vi "Tester.vi"() -> ()   [LabVIEW 2024]
uses:
  Shared Modules/CAN Commands Interpreter/CAN Frame Data.ctl
  Shared Modules/CAN Commands Interpreter/XNET Session Settings.ctl
  Type Definitions/Tester References.ctl
  Shared Modules/CAN Commands Interpreter/Command Values.ctl
  <vilib>/FPGAPlugInAG/PXI-7842R/niLvFpga_Open_PXI-7842R.vi
  <vilib>/rvi/interface/common/dynamic/niFpgaDynamicAddResources.vi
  <vilib>/FPGAPlugInAG/Dynamic/niLvFpga_Reset_Dynamic.vi
  Modules/Working Mode/Set Working Mode.vi
  Shared Modules/CAN Commands Interpreter/Target Sessions - Stop Session.vi
  Shared Modules/CAN Commands Interpreter/Target Sessions - Start Session.vi
  Shared Modules/CAN Commands Interpreter/Target Sessions - Clear Session.vi
  Shared Modules/CAN Commands Interpreter/Target Sessions - Initialize Output Session.vi
  Shared Modules/CAN Commands Interpreter/Target Sessions - Initialize Input Session.vi
  <vilib>/FPGAPlugInAG/Dynamic/niLvFpga_Run_Dynamic.vi
  <vilib>/Utility/error.llb/Error Cluster From Error Code.vi
  <vilib>/rvi/errors/niLvFpgaAdjustHostInterfaceError.vi
  <vilib>/FPGAPlugInAG/Dynamic/niLvFpga_Abort_Dynamic.vi
  <vilib>/FPGAPlugInAG/Dynamic/niLvFpga_Close_Dynamic.vi
  <vilib>/rvi/interface/nirviOpenFPGA/nirviOpenFPGA.xnode
  FPGA Bitfiles/tester-8880_FPGATarget_Tester-FPGA-Main_mAZV-GIAe8w.lvbitx
  <vilib>/rvi/interface/nirviMethod/nirviMethod.xnode
  <vilib>/rvi/interface/nirviReadWriteControl/nirviReadWriteControl.xnode
  <vilib>/rvi/interface/nirviCloseFPGA/nirviCloseFPGA.xnode
  Modules/Working Mode/Review Working Mode.vi
  Modules/Tester Internal Communication/References - Destroy.vi
  Modules/Tester Internal Communication/Queues - Destroy.vi
  Shared Modules/CAN Commands Interpreter/CAN Commands.lvlib
  Modules/UI/User Interface Control.lvlib
  Modules/Tester Internal Communication/Tester InterComm.lvlib
  Modules/Working Mode/Tester Working Mode.lvlib
  <vilib>/rvi/interface/Simulation/niFpgaSimulationCallBeginRW.vi
  <vilib>/rvi/errors/niLvFpgaMergeErrorWithErrorCode.vi
  <vilib>/FPGAPlugInAG/Dynamic/niLvFpga_StartFifo_Dynamic.vi
  <vilib>/FPGAPlugInAG/Dynamic/niLvFpga_ReadFifo_Dynamic.vi
  NiFpgaLv.dll
  <vilib>/FPGAPlugInAG/Dynamic/niLvFpga_StopFifo_Dynamic.vi
panel:
  in  "Tab Control":enum32{"Functionality", "Monitor", "Settings"}(tab)
  out "Throttle":dbl
  out "Crank Angle":dbl
  in  "Restart Communication":bool
  in  "STOP":bool
  out "ECU Connected":bool
  out "Messages Display":string
  in  "Working Mode":bool
  out "DO2 OUT":bool
  in  "DO1":bool
  out "DO1 OUT":bool
  in  "DO2":bool
  out "PWM Value":u8(slide) scale=0.0..100.0
  out "Voltage Value":dbl(slide) scale=0.0..10.0
  in  "PWM Out":u8 max=100 step=1
  in  "Voltage Out":dbl min=0.0 max=10.0 step=1.0
  in  "Read Speed":bool
  out "PWM Graph":sgl[](graph)
  out "Duty Cycle":dbl
  out "Frequency":dbl format="%#_6p"
  in  "Sine Enable/Disable":bool
  in  "Sinewave Out":u16(ring) items=["500 Hz", "1 KHz", "5 KHz"]
  out "Sinewave Graph":sgl[](graph)
  in  "PWM Enable/Disable":bool
  in  "V Enable/Disable":bool
  out "ECU Read Data":T1[][](array[typedef]) {"ID" format="%01x"; "Payload" format="%02x"}
  out "Current Working Mode":string
  in  "Commands File (CSV)":path=path "/home/admin/tester8880/CAN Commands.csv"
  out "XNET In Errors":errorcluster
  out "Event Errors":errorcluster
  out "UI Errors":errorcluster
  in  "Tester Sessions":T2[](array[typedef])=[{"Interface"="CAN2", "Frame List"=["ECU_Responses\nCAN Dataframes", "HeartBit\nCAN Dataframes", "Throttle\nCAN Dataframes", "Crank_Angle\nCAN Dataframes"], "Session ID"="", "Session Name"="Tester - Read ECU Responses"}, {"Interface"="CAN2", "Frame List"=["Tester_Requests\nCAN Dataframes"], "Session ID"="", "Session Name"="Tester - Write Requests"}, {"Interface"="CAN2", "Frame List"=["HeartBit\nCAN Dataframes"], "Session ID"="", "Session Name"="Tester - Write Heartbit"}]
  out "FPGA Errors":errorcluster
  # "Digital Outputs"
  # "Analog Outputs"
  # "Analog Inputs"
  # "Voltage"
  # "PWM"
  # "Sinewave"
  # "Motor Speed"
  # "Normal Values"
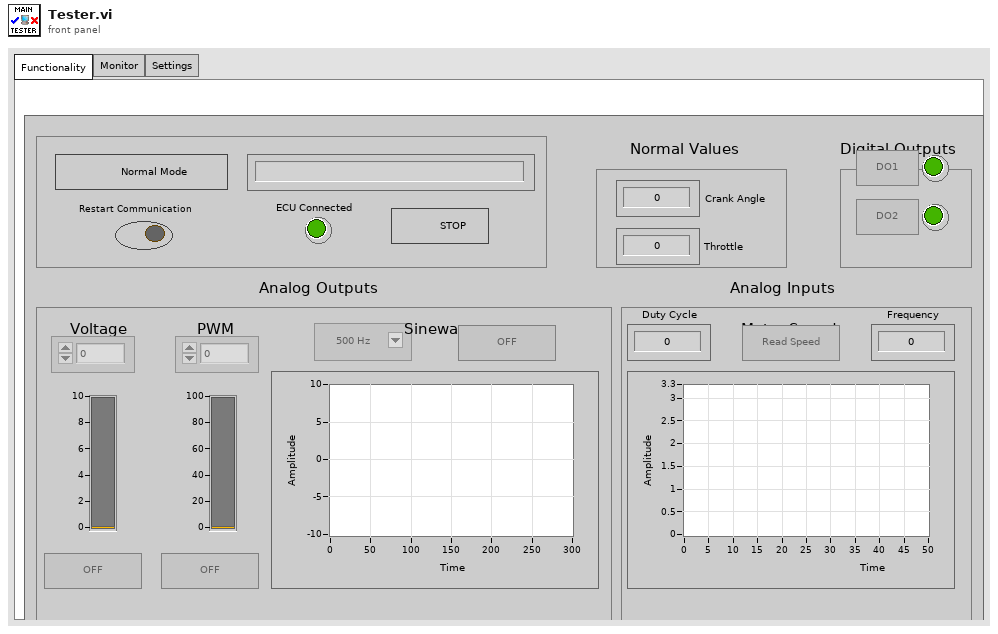
[diagram p1: front panel]
types:
  T1 = typedef "CAN Commands.lvlib/CAN Frame Data.ctl" = cluster{"Command":string, "XNET Frame":refnum<k21>, "Payload":u8[], "ID":u32, "Time Stamp":timestamp}
  T2 = typedef "CAN Commands.lvlib/XNET Session Settings.ctl" = cluster{"Interface":refnum<k21>, "Frame List":refnum<k21>[], "Session ID":refnum<k21>, "Session Name":string}
  T3 = typedef "Tester InterComm.lvlib/Tester References.ctl" = cluster{"This VI":cluster{"This VI":refnum<vi>}, "UI Menu":cluster{"Tab Control":refnum<vi>, "STOP":refnum<vi>, "Working Mode":refnum<vi>}, "Indicators":cluster{"Messages Display":refnum<vi>, "Voltage Value":refnum<vi>, "PWM Value":refnum<vi>, "PWM Graph":refnum<vi>, "Duty Cycle":refnum<vi>, "Frequency":refnum<vi>, "Sinewave Graph":refnum<vi>, "ECU Connected":refnum<vi>}, "Controls":cluster{"Read Speed":refnum<vi>, "Voltage Out":refnum<vi>, "V Enable/Disable":refnum<vi>, "PWM Enable/Disable":refnum<vi>, "PWM Out":refnum<vi>, "Sine Enable/Disable":refnum<vi>, "Sinewave Out":refnum<vi>, "DO1":refnum<vi>, "DO2":refnum<vi>}}
  T4 = cluster{"Tab Control":refnum<vi>, "STOP":refnum<vi>, "Working Mode":refnum<vi>}
  T5 = cluster{"Messages Display":refnum<vi>, "Voltage Value":refnum<vi>, "PWM Value":refnum<vi>, "PWM Graph":refnum<vi>, "Duty Cycle":refnum<vi>, "Frequency":refnum<vi>, "Sinewave Graph":refnum<vi>, "ECU Connected":refnum<vi>}
  T6 = cluster{"Read Speed":refnum<vi>, "Voltage Out":refnum<vi>, "V Enable/Disable":refnum<vi>, "PWM Enable/Disable":refnum<vi>, "PWM Out":refnum<vi>, "Sine Enable/Disable":refnum<vi>, "Sinewave Out":refnum<vi>, "DO1":refnum<vi>, "DO2":refnum<vi>}
  T7 = cluster{"Commands File (CSV)":path, "Tester Sessions":T2[], "References In":T3}
  T8 = typedef "CAN Commands.lvlib/Command Values.ctl" = cluster{"Command":string, "Value":dbl}
  T9 = cluster{"XNET Data[0]":T1, "XNET Data[1]":T1, "XNET Data[2]":T1, "XNET Data[3]":T1}
  T10 = cluster{"Commands[0]":T8, "Commands[1]":T8, "Commands[2]":T8, "Commands[3]":T8}
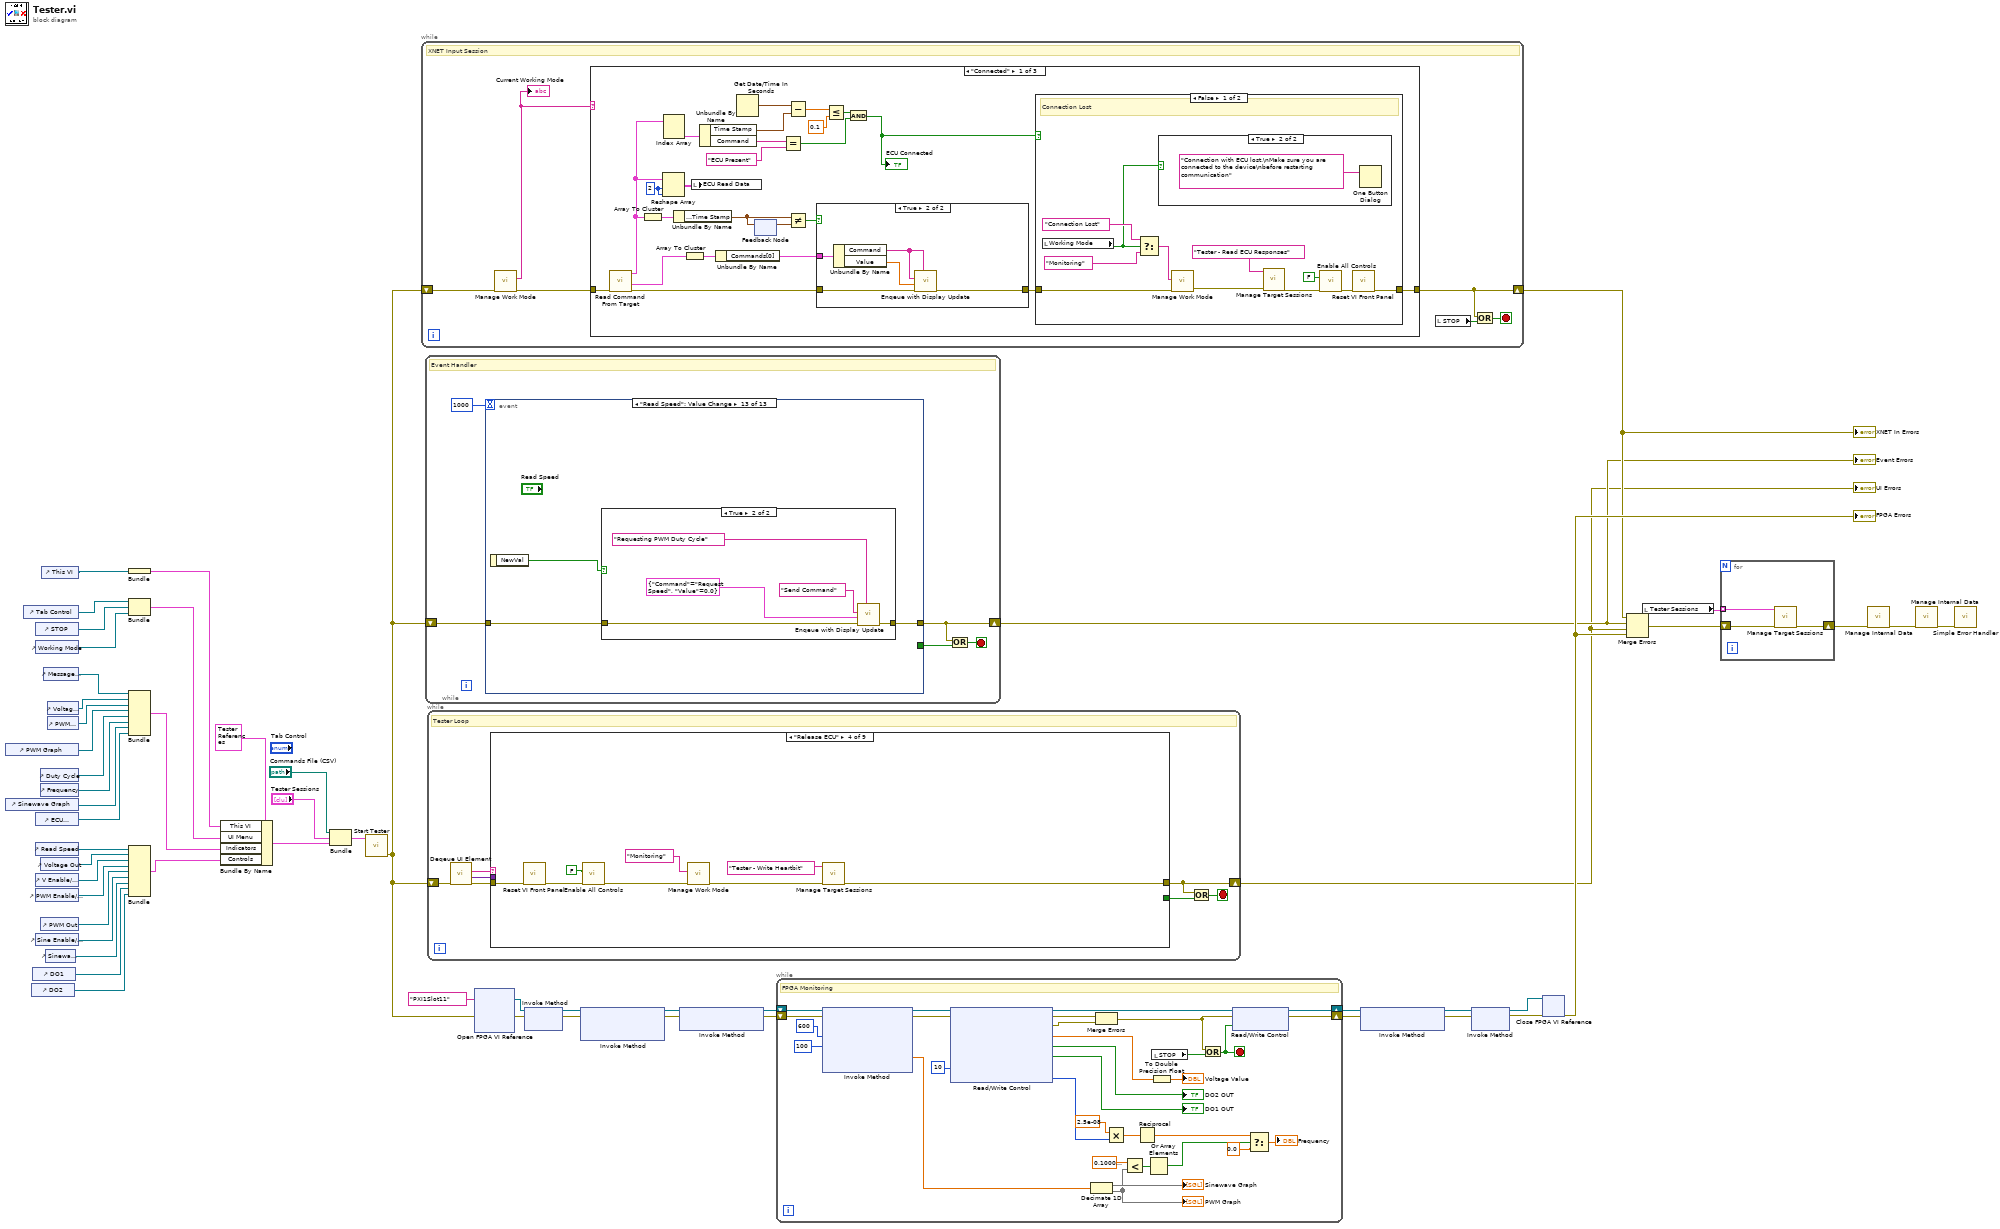
[diagram p0: block diagram]
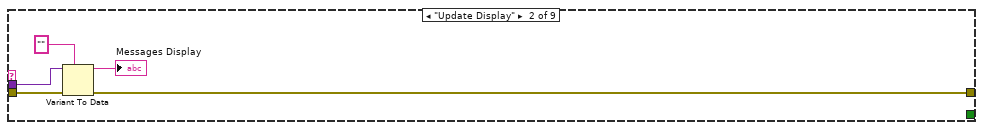
[diagram p3: hidden frame]
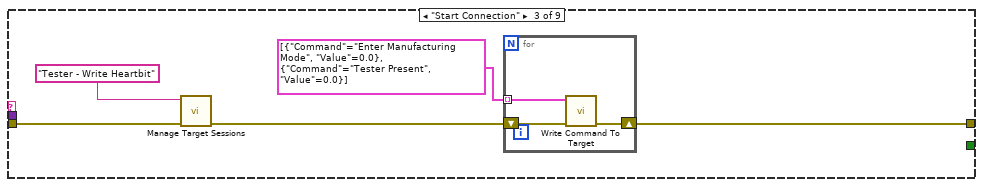
[diagram p4: hidden frame]
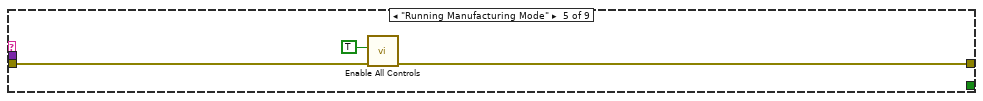
[diagram p5: hidden frame]
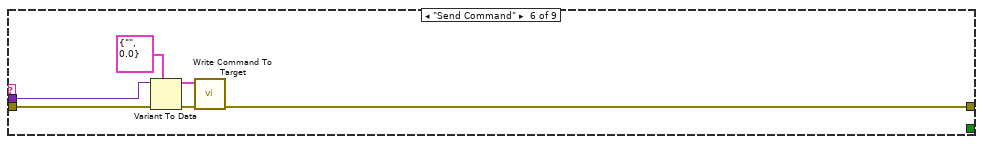
[diagram p6: hidden frame]
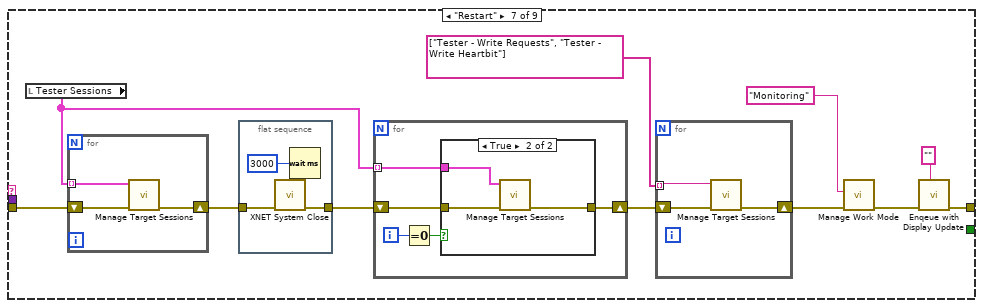
[diagram p7: hidden frame]
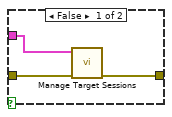
[diagram p8: hidden frame]
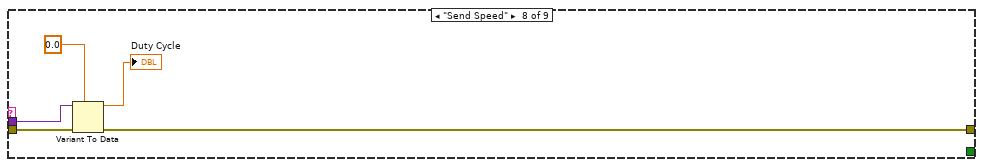
[diagram p9: hidden frame]
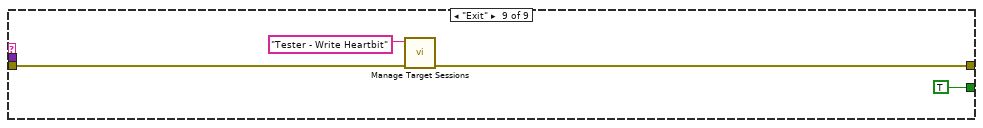
[diagram p10: hidden frame]
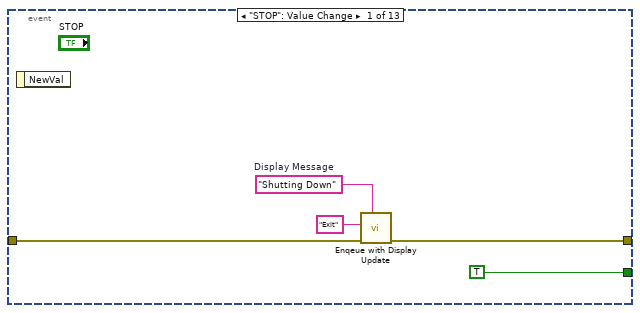
[diagram p11: hidden frame]
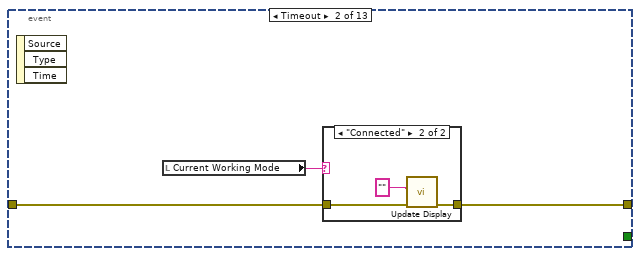
[diagram p12: hidden frame]
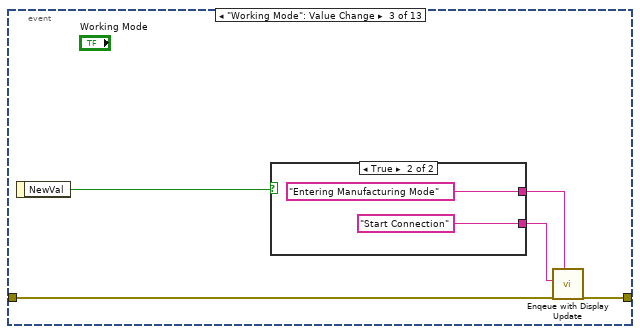
[diagram p14: hidden frame]
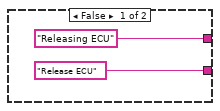
[diagram p15: hidden frame]
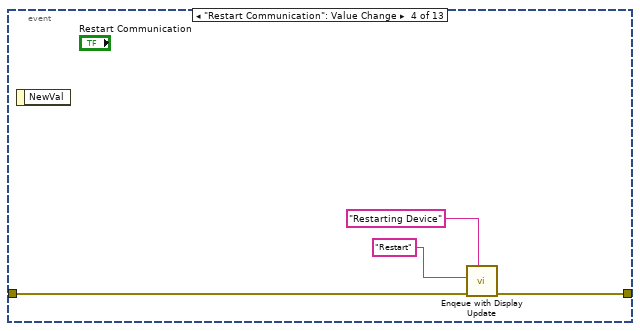
[diagram p16: hidden frame]
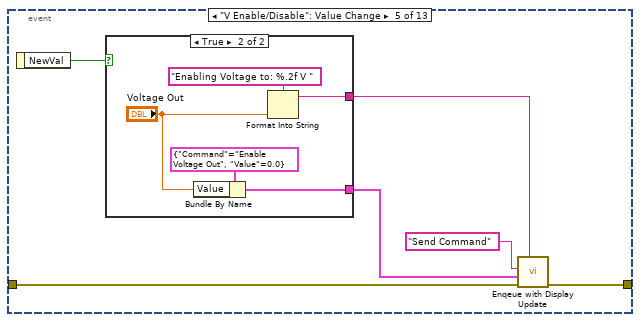
[diagram p17: hidden frame]
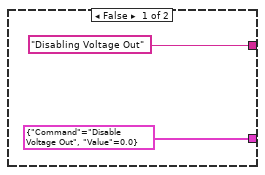
[diagram p18: hidden frame]
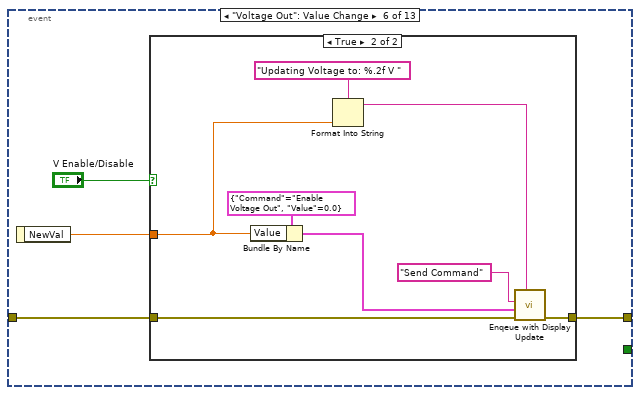
[diagram p19: hidden frame]
diagram:
  n1 = control-ref of="PWM Graph"() -> (w46:refnum<vi>)
  n2 = control-ref of="Sinewave Graph"() -> (w43:refnum<vi>)
  n3 = control-ref of="Tab Control"() -> (w41:refnum<vi>)
  n4 = control-ref of="DO2"() -> (w48:refnum<vi>)
  n5 = control-ref of="DO1"() -> (w49:refnum<vi>)
  n6 = control-ref of="STOP"() -> (w40:refnum<vi>)
  n7 = control-ref of="Working Mode"() -> (w39:refnum<vi>)
  n8 = control-ref of="ECU Connected"() -> (w42:refnum<vi>)
  n9 = control-ref of="Read Speed"() -> (w4:refnum<vi>)
  n10 = control-ref of="V Enable/Disable"() -> (w54:refnum<vi>)
  n11 = control-ref of="PWM Enable/Disable"() -> (w53:refnum<vi>)
  n12 = control-ref of="Sine Enable/Disable"() -> (w51:refnum<vi>)
  n13 = control-ref of="Duty Cycle"() -> (w45:refnum<vi>)
  n14 = control-ref of="Frequency"() -> (w44:refnum<vi>)
  n15 = control-ref of="Voltage Out"() -> (w55:refnum<vi>)
  n16 = control-ref of="PWM Out"() -> (w52:refnum<vi>)
  n17 = control-ref of="This VI"() -> (w37:refnum<vi>)
  n18 = control-ref of="Messages Display"() -> (w38:refnum<vi>)
  n19 = control-ref of="Sinewave Out"() -> (w50:refnum<vi>)
  n20 = control-ref of="Voltage Value"() -> (w34:refnum<vi>)
  n21 = control-ref of="PWM Value"() -> (w47:refnum<vi>)
  n22 = Bundle("This VI"=w37) -> (w36:cluster{"This VI":refnum<vi>})  [unwired: 1 in]
  n23 = Bundle("Tab Control"=w41, "STOP"=w40, "Working Mode"=w39) -> (w33:T4)  [unwired: 1 in]
  n24 = Bundle("Messages Display"=w38, "Voltage Value"=w34, "PWM Value"=w47, "PWM Graph"=w46, "Duty Cycle"=w45, "Frequency"=w44, "Sinewave Graph"=w43, "ECU Connected"=w42) -> (w35:T5)  [unwired: 1 in]
  n25 = Bundle("Read Speed"=w4, "Voltage Out"=w55, "V Enable/Disable"=w54, "PWM Enable/Disable"=w53, "PWM Out"=w52, "Sine Enable/Disable"=w51, "Sinewave Out"=w50, "DO1"=w49, "DO2"=w48) -> (w1:T6)  [unwired: 1 in]
  n26 = Bundle By Name(cluster=T3 {"This VI"={"This VI"=refnum}, "UI Menu"={"Tab Control"=refnum, "STOP"=refnum, "Working Mode"=refnum}, "Indicators"={"Messages Display"=refnum, "Voltage Value"=refnum, "PWM Value"=refnum, "PWM Graph"=refnum, "Duty Cycle"=refnum, "Frequency"=refnum, "Sinewave Graph"=refnum, "ECU Connected"=refnum}, "Controls"={"Read Speed"=refnum, "Voltage Out"=refnum, "V Enable/Disable"=refnum, "PWM Enable/Disable"=refnum, "PWM Out"=refnum, "Sine Enable/Disable"=refnum, "Sinewave Out"=refnum, "DO1"=refnum, "DO2"=refnum}} ("References In"), "This VI"=w36, "UI Menu"=w33, "Indicators"=w35, "Controls"=w1) -> (w3:T3)
  n27 = Bundle("Commands File (CSV)"="Commands File (CSV)", "Tester Sessions"="Tester Sessions", "References In"=w3) -> (w2:T7)  [unwired: 1 in]
  n28 = call "Start Tester.vi"("Tester Settings"=w2) -> ("error out"=w15:errorcluster)  [unwired: 10 in]
  n29 = while {
    shift-right: [w56] -> w8
    shift-left: w15 -> [w60]
    stop <- w57 stop-if-true
    # "XNET Input Session"
    n30 = call-poly "Manage Work Mode.vi"("error in"=w60) -> ("error out"=w59:errorcluster, "Message"=w58:string)  [unwired: 8 in, 1 out]
    "Current Working Mode" <- w58
    n31 = case shown="\"Connected\"" w58 {
      tunnel: [w71 w121 w128] -> w56
      tunnel: w59 -> [w70 w119 w128]
      frame "Connected" {
        w81 = 2 ("dimension size")
        n32 = call "Read Command From Target.vi"("error in"=w70) -> ("error out"=w69:errorcluster, "Commands"=w68:T8[], "XNET Data"=w67:T1[])  [unwired: 7 in, 1 out]
        n33 = Array To Cluster(array=w67) -> (cluster=w82:T9)
        n34 = Reshape Array(w67, w81, w81) -> (w63:T1[][])
        n35 = Index Array(array=w67) -> (element #2=w64:T1)  [unwired: 2 in, 1 out]
        n36 = Unbundle By Name(w82) -> ("XNET Data[0].Time Stamp"=w83:timestamp)
        n37 = Array To Cluster(array=w68) -> (cluster=w80:T10)
        n38 = local write "ECU Read Data"(w63) -> ()
        n39 = Unbundle By Name(w64) -> ("Time Stamp"=w66:timestamp, "Command"=w65:string)
        n40 = Unbundle By Name(w80) -> ("Commands[0]"=w79:T8)
        n41 = Get Date/Time In Seconds() -> (seconds since 1Jan1904=w78:timestamp)
        n42 = feedback #1() -> (w84:timestamp)  [unwired: 1 in]
        n43 = feedback-in #1(w83) -> ()
        n44 = Equal?(x=w65, y="ECU Present") -> (x = y?=w73:bool)
        n45 = Not Equal?(x=w83, y=w84) -> (x != y?=w85:bool)
        n46 = Subtract(x=w78, y=w66) -> (x-y=w77:dbl)
        n47 = case shown="True" w85 {
          tunnel: w69 -> [w99 w104]
          tunnel: [w99 w103] -> w72
          tunnel: w79 -> [_ w100]
          frame False {
          }
          frame True {
            n48 = Unbundle By Name(w100) -> ("Command"=w102:string, "Value"=w101:dbl)
            n49 = call "Enqeue with Display Update.vi"("Display Message"=w102, "error in"=w104, "Data"=w101, "Message"=w102) -> ("error out"=w103:errorcluster)  [unwired: 7 in]
          }
        }
        n50 = Less Or Equal?(x=w77, y=0.1) -> (x <= y?=w75:bool)
        n51 = And(x=w75, y=w73) -> (x .and. y?=w62:bool)
        "ECU Connected" <- w62
        n52 = case shown="False" w62 {
          tunnel: [w86 w98] -> w71
          tunnel: w72 -> [w96 w98]
          frame False {
            # "Connection Lost"
            n53 = local read "Working Mode"() -> (w90:bool)
            n54 = Select(t="Connection Lost" ("Message"), s=w90, f="Monitoring" ("Message")) -> (s? t:f=w91:string)
            n55 = case shown="True" w90 {
              frame False {
              }
              frame True {
                n56 = One Button Dialog(message="Connection with ECU lost.\nMake sure you are connected to the device\nbefore restarting communication") -> ()  [unwired: 1 in, 1 out]
              }
            }
            n57 = call-poly "Manage Work Mode.vi"("error in"=w96, "Message"=w91) -> ("error out"=w95:errorcluster)  [unwired: 9 in]
            n58 = call-poly "Manage Target Sessions.vi"("error in"=w95, "Session Name"="Tester - Read ECU Responses") -> ("error out"=w88:errorcluster)  [unwired: 9 in]
            n59 = call "Enable All Controls.vi"("error in"=w88, "Enable Controls"=FALSE) -> ("error out"=w87:errorcluster)  [unwired: 9 in]
            n60 = call "Reset VI Front Panel.vi"("error in"=w87) -> ("error out"=w86:errorcluster)  [unwired: 10 in]
          }
          frame True {
          }
        }
      }
      frame "Monitoring", Default {
        w123 = 2 ("dimension size")
        n61 = call "Read Command From Target.vi"("error in"=w119) -> ("error out"=w118:errorcluster, "Values"=w109:dbl[], "XNET Data"=w114:T1[])  [unwired: 7 in, 1 out]
        n62 = Array To Cluster(array=w114) -> (cluster=w113:T9)
        n63 = Index Array(array=w109, index #1=3 ("index"), index #2=2 ("index")) -> (element #1=→"Crank Angle":dbl, element #2=→"Throttle":dbl)
        n64 = Reshape Array(w114, w123, w123) -> (→"ECU Read Data":T1[][])
        n65 = Unbundle By Name(w113) -> ("XNET Data[0].Command"=w112:string, "XNET Data[1].Command"=w116:string)
        n66 = Equal?(x="Running Manufacturing Mode" ("y"), y=w112) -> (x = y?=w120:bool)
        n67 = Equal?(x=w116, y="ECU Present") -> (x = y?=w110:bool)
        n68 = And(x=w120, y=w110) -> (x .and. y?=w111:bool)
        n69 = case shown="False" w111 {
          tunnel: [w124 w126] -> w121
          tunnel: w118 -> [w124 w125]
          frame False {
          }
          frame True {
            # "ECU Found"
            n70 = call-poly "Manage Work Mode.vi"("error in"=w125, "Message"="Connected") -> ("error out"=w126:errorcluster)  [unwired: 9 in]
          }
        }
      }
      frame "Connection Lost" {
      }
    }
    n71 = local read "STOP"() -> (w61:bool)
    n72 = Or(x=w56, y=w61) -> (x .or. y?=w57:bool)
  }
  "XNET In Errors" <- w8
  n73 = while {
    shift-right: [w130] -> w7
    shift-left: w15 -> [w132]
    stop <- w131 stop-if-true
    # "Event Handler"
    n74 = event shown="[12] \"Read Speed\": Value Change" {
      selector: _ -> [_ _ _ _ _ _ _ _ _ _ _ _ _]
      dyn-events: _ -> [_ _ _ _ _ _ _ _ _ _ _ _ _]
      timeout: 1000 -> [_ _ _ _ _ _ _ _ _ _ _ _ _]
      tunnel: [TRUE _ _ _ _ _ _ _ _ _ _ _ _] -> w133
      tunnel: [w134 w141 w148 w157 w163 w173 w185 w214 w222 w233 w249 w261 w268] -> w130
      tunnel: w132 -> [w136 w140 w147 w156 w164 w172 w189 w215 w219 w235 w250 w260 w267]
      event "STOP": Value Change {
        w135 = "Shutting Down"  # Display Message
        n75 = event-data() -> ()  [unwired: 1 in, 1 out]
        n76 = call "Enqeue with Display Update.vi"("Display Message"=w135, "error in"=w136, "Message"="Exit") -> ("error out"=w134:errorcluster)  [unwired: 8 in]
      }
      event Timeout {
        n77 = event-data() -> ()  [unwired: 1 in, 3 out]
        n78 = local read "Current Working Mode"() -> (w139:string)
        n79 = case shown="\"Connected\"" w139 {
          tunnel: [w142 w145] -> w141
          tunnel: w140 -> [w142 w144]
          frame "", Default {
          }
          frame "Connected" {
            n80 = call "Update Display.vi"("error in"=w144, "Display Message"="") -> ("error out"=w145:errorcluster)  [unwired: 9 in]
          }
        }
      }
      event "Working Mode": Value Change {
        n81 = event-data() -> ("NewVal"=w146:bool)  [unwired: 1 in]
        n82 = case shown="True" w146 {
          tunnel: ["Releasing ECU" ("Message") "Entering Manufacturing Mode" ("Message")] -> w150
          tunnel: ["Release ECU" ("Message") "Start Connection" ("Message")] -> w149
          frame False {
          }
          frame True {
          }
        }
        n83 = call "Enqeue with Display Update.vi"("Display Message"=w150, "error in"=w147, "Message"=w149) -> ("error out"=w148:errorcluster)  [unwired: 8 in]
      }
      event "Restart Communication": Value Change {
        n84 = event-data() -> ()  [unwired: 1 in, 1 out]
        n85 = call "Enqeue with Display Update.vi"("Display Message"="Restarting Device", "error in"=w156, "Message"="Restart") -> ("error out"=w157:errorcluster)  [unwired: 8 in]
      }
      event "V Enable/Disable": Value Change {
        n86 = event-data() -> ("NewVal"=w161:bool)  [unwired: 1 in]
        n87 = case shown="True" w161 {
          tunnel: ["Disabling Voltage Out" ("Message") w170] -> w162
          tunnel: [T8 {"Command"="Disable Voltage Out", "Value"=0.0} ("Command Data") w167] -> w160
          frame False {
          }
          frame True {
            n88 = Bundle By Name(cluster=T8 {"Command"="Enable Voltage Out", "Value"=0.0} ("Command Data"), "Value"="Voltage Out") -> (w167:T8)
            n89 = Format Into String(format string="Enabling Voltage to: %.2f V " ("Message"), "Voltage Out") -> (resulting string=w170:string)  [unwired: 2 in, 1 out]
          }
        }
        n90 = call "Enqeue with Display Update.vi"("Display Message"=w162, "error in"=w164, "Data"=w160, "Message"="Send Command") -> ("error out"=w163:errorcluster)  [unwired: 7 in]
      }
      event "Voltage Out": Value Change {
        n91 = event-data() -> ("NewVal"=w174:dbl)  [unwired: 1 in]
        n92 = case shown="True" "V Enable/Disable" {
          tunnel: w174 -> [_ w180]
          tunnel: [w176 w179] -> w173
          tunnel: w172 -> [w176 w178]
          frame False {
          }
          frame True {
            n93 = Bundle By Name(cluster=T8 {"Command"="Enable Voltage Out", "Value"=0.0} ("Command Data"), "Value"=w180) -> (w181:T8)
            n94 = Format Into String(format string="Updating Voltage to: %.2f V " ("Message"), w180) -> (resulting string=w182:string)  [unwired: 2 in, 1 out]
            n95 = call "Enqeue with Display Update.vi"("Display Message"=w182, "error in"=w178, "Data"=w181, "Message"="Send Command") -> ("error out"=w179:errorcluster)  [unwired: 7 in]
          }
        }
      }
      event "PWM Enable/Disable": Value Change {
        n96 = event-data() -> ("NewVal"=w187:bool)  [unwired: 1 in]
        n97 = Not(x=w187) -> (.not. x?=w188:bool)
        n98 = call "Enable PWM Out.vi"("error in"=w189, "Enable PWM Out"=w188) -> ("error out"=w186:errorcluster)  [unwired: 9 in]
        n99 = case shown="True" w187 {
          tunnel: w186 -> [w194 w196]
          tunnel: [w193 w198] -> w185
          frame False {
            n100 = call "Enqeue with Display Update.vi"("Display Message"="Disabling PWM", "error in"=w194, "Data"=T8 {"Command"="Disable PWM", "Value"=0.0} ("Command Data"), "Message"="Send Command") -> ("error out"=w193:errorcluster)  [unwired: 7 in]
          }
          frame True {
            n101 = Format Into String(format string="Enabling PWM to %d of Duty Cycle", "PWM Out") -> (resulting string=w195:string)  [unwired: 2 in, 1 out]
            n102 = for {
              tunnel: T8[] [{"Command"="Configure PWM", "Value"=0.0}, {"Command"="Enable PWM", "Value"=0.0}] -> [w205] mode=indexing
              shift-right: [w204] -> w198
              shift-left: w196 -> [w202]
              tunnel: "PWM Out" -> [w203]
              tunnel: w195 -> [w201]
              n103 = Bundle By Name(cluster=w205, "Value"=w203) -> (w206:T8)
              n104 = call "Enqeue with Display Update.vi"("Display Message"=w201, "error in"=w202, "Data"=w206, "Message"="Send Command") -> ("error out"=w204:errorcluster)  [unwired: 7 in]
            }
          }
        }
      }
      event "PWM Out": Value Change {
        n105 = event-data() -> ("NewVal"=w213:u8)  [unwired: 1 in]
        "PWM Value" <- w213
        n106 = Bundle By Name(cluster=T8 {"Command"="Configure PWM", "Value"=0.0} ("Command Data"), "Value"=w213) -> (w209:T8)
        n107 = Format Into String(format string="Updating PWM to %d of Duty Cycle", w213) -> (resulting string=w211:string)  [unwired: 2 in, 1 out]
        n108 = call "Enqeue with Display Update.vi"("Display Message"=w211, "error in"=w215, "Data"=w209, "Message"="Send Command") -> ("error out"=w214:errorcluster)  [unwired: 7 in]
      }
      event "Sine Enable/Disable": Value Change {
        n109 = event-data() -> ("NewVal"=w220:bool)  [unwired: 1 in]
        n110 = Not(x=w220) -> (.not. x?=w221:bool)
        n111 = call "Enable Sinewave Out Value.vi"("error in"=w219, "Enable Sinewave Out"=w221) -> ("error out"=w217:errorcluster)  [unwired: 9 in]
        n112 = case shown="True" w220 {
          tunnel: ["Disabling Sinewave" "Enabling Sinewave"] -> w223
          tunnel: [T8 {"Command"="Disable Sinewave", "Value"=0.0} ("Command Data") w227] -> w218
          frame False {
          }
          frame True {
            n113 = Bundle By Name(cluster=T8 {"Command"="Enable Sinewave", "Value"=0.0} ("Command Data"), "Value"="Sinewave Out") -> (w227:T8)
          }
        }
        n114 = call "Enqeue with Display Update.vi"("Display Message"=w223, "error in"=w217, "Data"=w218, "Message"="Send Command") -> ("error out"=w222:errorcluster)  [unwired: 7 in]
      }
      event "Sinewave Out": Value Change {
        n115 = event-data() -> ("NewVal"=w234:u16)  [unwired: 1 in]
        n116 = Bundle By Name(cluster=T8 {"Command"="Configure Sinewave", "Value"=0.0} ("Command Data"), "Value"=w234) -> (w231:T8)
        n117 = case shown="0, Default" w234 {
          tunnel: [u16 500 ("NewVal") u16 1 ("NewVal") u16 5 ("NewVal")] -> w238
          tunnel: ["Hz" ("input 2") "KHz" ("input 2") "KHz" ("input 2")] -> w237
          frame 0, Default {
          }
          frame 1 {
          }
          frame 2 {
          }
        }
        n118 = Format Into String(format string="Configuring Waveform to: %d %s" ("Message"), w238, w237) -> (resulting string=w232:string)  [unwired: 2 in, 1 out]
        n119 = call "Enqeue with Display Update.vi"("Display Message"=w232, "error in"=w235, "Data"=w231, "Message"="Send Command") -> ("error out"=w233:errorcluster)  [unwired: 7 in]
      }
      event "DO1": Value Change {
        n120 = event-data() -> ("NewVal"=w251:bool)  [unwired: 1 in]
        n121 = case shown="True" w251 {
          tunnel: ["Disabling DO1" "Enabling DO1"] -> w248
          tunnel: [T8 {"Command"="DO1 OFF", "Value"=0.0} ("Command Data") T8 {"Command"="DO1 ON", "Value"=1.0} ("Command Data")] -> w247
          frame False {
          }
          frame True {
          }
        }
        n122 = call "Enqeue with Display Update.vi"("Display Message"=w248, "error in"=w250, "Data"=w247, "Message"="Send Command") -> ("error out"=w249:errorcluster)  [unwired: 7 in]
      }
      event "DO2": Value Change {
        n123 = event-data() -> ("NewVal"=w259:bool)  [unwired: 1 in]
        n124 = case shown="False" w259 {
          tunnel: ["Disabling DO2" "Enabling DO2"] -> w258
          tunnel: [T8 {"Command"="DO2 OFF", "Value"=0.0} ("Command Data") T8 {"Command"="DO2 ON", "Value"=1.0} ("Command Data")] -> w257
          frame False {
          }
          frame True {
          }
        }
        n125 = call "Enqeue with Display Update.vi"("Display Message"=w258, "error in"=w260, "Data"=w257, "Message"="Send Command") -> ("error out"=w261:errorcluster)  [unwired: 7 in]
      }
      event "Read Speed": Value Change {
        n126 = event-data() -> ("NewVal"=w266:bool)  [unwired: 1 in]
        n127 = case shown="True" w266 {
          tunnel: [w269 w273] -> w268
          tunnel: w267 -> [w269 w272]
          frame False {
          }
          frame True {
            n128 = call "Enqeue with Display Update.vi"("Display Message"="Requesting PWM Duty Cycle", "error in"=w272, "Data"=T8 {"Command"="Request Speed", "Value"=0.0} ("Command Data"), "Message"="Send Command") -> ("error out"=w273:errorcluster)  [unwired: 7 in]
          }
        }
      }
    }
    n129 = Or(x=w130, y=w133) -> (x .or. y?=w131:bool)
  }
  "Event Errors" <- w7
  n130 = while {
    shift-right: [w279] -> w6
    shift-left: w15 -> [w278]
    stop <- w280 stop-if-true
    # "Tester Loop"
    n131 = call "Deqeue UI Element.vi"("error in"=w278) -> ("error out"=w277:errorcluster, "Data"=w275:variant, "Message"=w276:string)  [unwired: 8 in]
    n132 = case shown="\"Release ECU\"" w276 {
      tunnel: w275 -> [_ w285 _ _ _ w308 _ w344 _]
      tunnel: w277 -> [w282 w287 w292 w297 w306 w309 w318 w346 w352]
      tunnel: [w282 w286 w291 w302 w305 w307 w315 w345 w351] -> w279
      tunnel: [_ _ _ _ _ _ _ _ TRUE] -> w281
      frame "", Default {
      }
      frame "Update Display" {
        n133 = Variant To Data(error in=w287, type="", Variant=w285) -> (data=→"Messages Display":string, error out=w286:errorcluster)
      }
      frame "Start Connection" {
        n134 = call-poly "Manage Target Sessions.vi"("error in"=w292, "Session Name"="Tester - Write Heartbit") -> ("error out"=w289:errorcluster)  [unwired: 9 in]
        n135 = for {
          shift-right: [w294] -> w291
          shift-left: w289 -> [w295]
          tunnel: T8[] [{"Command"="Enter Manufacturing Mode", "Value"=0.0}, {"Command"="Tester Present", "Value"=0.0}] -> [w293] mode=indexing
          n136 = call "Write Command To Target.vi"("error out"=w295, "Command"=w293) -> ("error out"=w294:errorcluster)  [unwired: 9 in]
        }
      }
      frame "Release ECU" {
        n137 = call "Reset VI Front Panel.vi"("error in"=w297) -> ("error out"=w296:errorcluster)  [unwired: 10 in]
        n138 = call "Enable All Controls.vi"("error in"=w296, "Enable Controls"=FALSE) -> ("error out"=w299:errorcluster)  [unwired: 9 in]
        n139 = call-poly "Manage Work Mode.vi"("error in"=w299, "Message"="Monitoring") -> ("error out"=w300:errorcluster)  [unwired: 9 in]
        n140 = call-poly "Manage Target Sessions.vi"("error in"=w300, "Session Name"="Tester - Write Heartbit") -> ("error out"=w302:errorcluster)  [unwired: 9 in]
      }
      frame "Running Manufacturing Mode" {
        n141 = call "Enable All Controls.vi"("error in"=w306, "Enable Controls"=TRUE) -> ("error out"=w305:errorcluster)  [unwired: 9 in]
      }
      frame "Send Command" {
        n142 = Variant To Data(error in=w309, type=T8 {"Command"="", "Value"=0.0} ("Command Data"), Variant=w308) -> (data=w311:T8, error out=w310:errorcluster)
        n143 = call "Write Command To Target.vi"("error out"=w310, "Command"=w311) -> ("error out"=w307:errorcluster)  [unwired: 9 in]
      }
      frame "Restart" {
        n144 = local read "Tester Sessions"() -> (w323:T2[])
        n145 = for {
          shift-right: [w343] -> w321
          shift-left: w318 -> [w342]
          tunnel: w323 -> [w341] mode=indexing
          n146 = call-poly "Manage Target Sessions.vi"("error in"=w342, "XNET Session"=w341) -> ("error out"=w343:errorcluster)  [unwired: 9 in]
        }
        n147 = flat-sequence {
          tunnel: w321 -> [w326]
          tunnel: [w325] -> w320
          frame #0 {
            n148 = call <vilib>:"XNET System Close.vi"("error in (no error)"=w326) -> ("error out"=w325:errorcluster)  [unwired: 14 in]
            n149 = Wait (ms)(milliseconds to wait=u32 3000) -> ()  [unwired: 1 out]
          }
        }
        n150 = for {
          shift-right: [w334] -> w322
          shift-left: w320 -> [w333]
          tunnel: w323 -> [w332] mode=indexing
          i -> [w330]
          n151 = Equal To 0?(x=w330) -> (x = 0?=w331:bool)
          n152 = case shown="True" w331 {
            tunnel: [w336 w340] -> w334
            tunnel: w333 -> [w337 w339]
            tunnel: w332 -> [w335 w338]
            frame False {
              n153 = call-poly "Manage Target Sessions.vi"("error in"=w337, "XNET Session Resouces"=w335) -> ("error out"=w336:errorcluster)  [unwired: 9 in]
            }
            frame True {
              n154 = call-poly "Manage Target Sessions.vi"("error in"=w339, "XNET Session Resouces"=w338) -> ("error out"=w340:errorcluster)  [unwired: 9 in]
            }
          }
        }
        n155 = for {
          shift-right: [w329] -> w317
          shift-left: w322 -> [w328]
          tunnel: string[] ["Tester - Write Requests", "Tester - Write Heartbit"] -> [w327] mode=indexing
          n156 = call-poly "Manage Target Sessions.vi"("error in"=w328, "Session Name"=w327) -> ("error out"=w329:errorcluster)  [unwired: 9 in]
        }
        n157 = call-poly "Manage Work Mode.vi"("error in"=w317, "Message"="Monitoring") -> ("error out"=w314:errorcluster)  [unwired: 9 in]
        n158 = call "Enqeue with Display Update.vi"("Display Message"="", "error in"=w314) -> ("error out"=w315:errorcluster)  [unwired: 9 in]
      }
      frame "Send Speed" {
        n159 = Variant To Data(error in=w346, type=0.0 ("Duty Cycle"), Variant=w344) -> (data=→"Duty Cycle":dbl, error out=w345:errorcluster)
      }
      frame "Exit" {
        n160 = call-poly "Manage Target Sessions.vi"("error in"=w352, "Session Name"="Tester - Write Heartbit") -> ("error out"=w351:errorcluster)  [unwired: 9 in]
      }
    }
    n161 = Or(x=w279, y=w281) -> (x .or. y?=w280:bool)
  }
  "UI Errors" <- w6
  n162 = xnode "Open FPGA VI Reference"("error in"=w15, "resource name"=tag "PXI1Slot11") -> ("FPGA VI Reference Out"=w18:refnum<k20>, "error out"=w25:errorcluster)
  n163 = xnode "Invoke Method"("FPGA VI Reference In"=w18, "error in"=w25) -> ("FPGA VI Reference Out"=w16:refnum<k20>, "error out"=w24:errorcluster)
  n164 = xnode "Invoke Method"("FPGA VI Reference In"=w16, "error in"=w24) -> ("FPGA VI Reference Out"=w13:refnum<k20>, "error out"=w17:errorcluster)  [unwired: 1 in]
  n165 = xnode "Invoke Method"("FPGA VI Reference In"=w13, "error in"=w17) -> ("FPGA VI Reference Out"=w12:refnum<k20>, "error out"=w14:errorcluster)
  n166 = while {
    shift-right: [w383] -> w10
    shift-left: w12 -> [w370]
    shift-right: [w382] -> w23
    shift-left: w14 -> [w379]
    stop <- w380 stop-if-true
    # "FPGA Monitoring"
    n167 = xnode "Invoke Method"("FPGA VI Reference In"=w370, "error in"=w379, "Number of Elements"=u32 600, "Timeout (ms)"=100) -> ("FPGA VI Reference Out"=w369:refnum<k20>, "error out"=w371:errorcluster, "Data"=w366:sgl[])  [unwired: 1 out]
    n168 = xnode "Read/Write Control"("FPGA VI Reference In"=w369, "error in"=w371, "Signal Sample Rate"=u32 10) -> ("FPGA VI Reference Out"=w377:refnum<k20>, "error out"=w378:errorcluster, "FPGA error"=w374:errorcluster, "ReadVoltageOut"=w376:sgl, "ReadDO1"=→"DO2 OUT":bool, "ReadDO2"=→"DO1 OUT":bool, "Measured Period (Ticks)"=w360:u32)
    n169 = Decimate 1D Array(w366) -> (→"Sinewave Graph":sgl[], w361:sgl[])
    "PWM Graph" <- w361
    n170 = Merge Errors(w378, w374) -> (w375:errorcluster)
    n171 = Multiply(x=2.5e-08, y=w360) -> (x*y=w372:dbl)
    n172 = Less?(x=sgl 0.1, y=w361) -> (x < y?=w357:bool[])
    n173 = Reciprocal(x=w372) -> (1/x=w354:dbl)
    n174 = Or Array Elements(Boolean array=w357) -> (logical OR=w355:bool)
    n175 = To Double Precision Float(number=w376) -> (double precision float=→"Voltage Value":dbl)
    n176 = local read "STOP"() -> (w381:bool)
    n177 = Or(x=w375, y=w381) -> (x .or. y?=w380:bool)
    n178 = xnode "Read/Write Control"("FPGA VI Reference In"=w377, "error in"=w375, "STOP FPGA"=w380) -> ("FPGA VI Reference Out"=w383:refnum<k20>, "error out"=w382:errorcluster)
    n179 = Select(t=w354, s=w355, f=0.0) -> (s? t:f=→"Frequency":dbl)
  }
  n180 = xnode "Invoke Method"("FPGA VI Reference In"=w10, "error in"=w23) -> ("FPGA VI Reference Out"=w9:refnum<k20>, "error out"=w11:errorcluster)
  n181 = xnode "Invoke Method"("FPGA VI Reference In"=w9, "error in"=w11) -> ("FPGA VI Reference Out"=w22:refnum<k20>, "error out"=w21:errorcluster)
  n182 = xnode "Close FPGA VI Reference"("FPGA VI Reference In"=w22, "error in"=w21) -> ("error out"=w20:errorcluster)
  "FPGA Errors" <- w20
  n183 = Merge Errors(w8, w7, w6, w20) -> (w32:errorcluster)
  n184 = local read "Tester Sessions"() -> (w30:T2[])
  n185 = for {
    shift-right: [w385] -> w26
    shift-left: w32 -> [w386]
    tunnel: w30 -> [w384] mode=indexing
    n186 = call-poly "Manage Target Sessions.vi"("error in"=w386, "XNET Session"=w384) -> ("error out"=w385:errorcluster)  [unwired: 9 in]
  }
  n187 = call-poly "Manage Internal Data.vi"("error in"=w26) -> ("error out"=w28:errorcluster)  [unwired: 10 in]
  n188 = call-poly "Manage Internal Data.vi"("error in"=w28) -> ("error out"=w27:errorcluster)  [unwired: 10 in]
  n189 = call <vilib>:"Simple Error Handler.vi"("error in (no error)"=w27) -> ()  [unwired: 4 in, 5 out]
